vi "rightJustifyColumn.vi"(8 "error in (no error)":errorcluster, 11 "ScriptEditorV2 in":refnum<class "ScriptEditorV2.lvclass">) -> (0 "error out":errorcluster, 3 "ScriptEditorV2 out":refnum<class "ScriptEditorV2.lvclass">)   [LabVIEW 2011, in "Views.lvlib" / "ScriptEditor.lvlib" / "ScriptEditorV2.lvclass"]
uses:
  ScriptEditorV2.lvclass
  ScriptEditorV2.lvclass/ScriptEditorV2.ctl
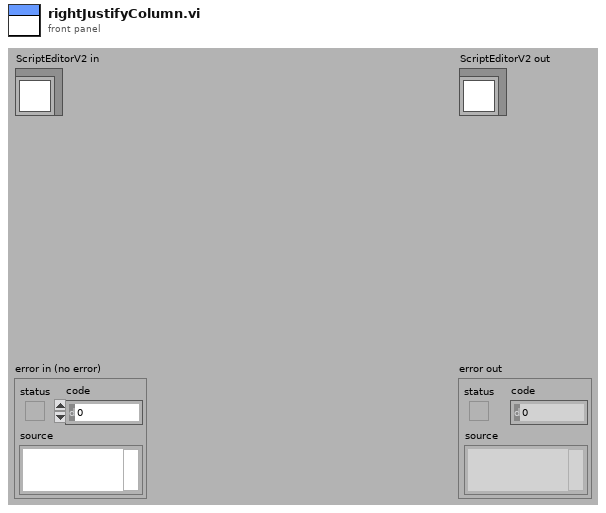
[diagram p1: front panel]
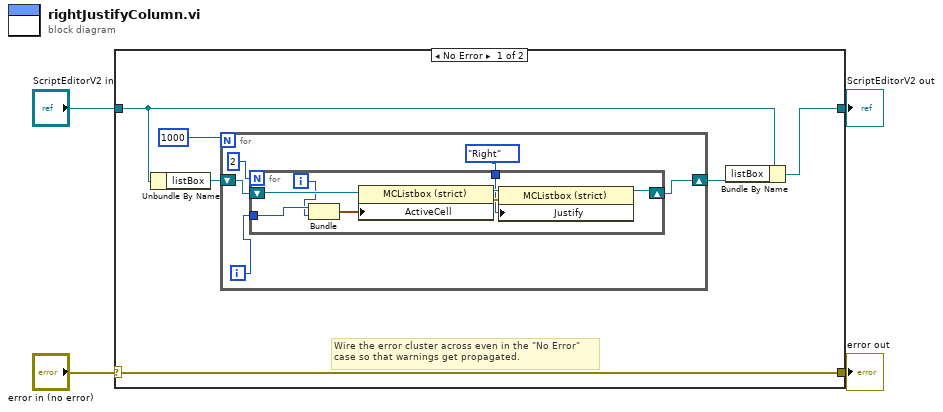
[diagram p0: block diagram]
diagram:
  n1 = case shown="No Error" "error in (no error)" {
    selector: "error in (no error)" -> [w10 w25]
    tunnel: [w10 w25] -> w3
    tunnel: [w6 w24] -> w1
    tunnel: "ScriptEditorV2 in" -> [w7 w24]
    frame No Error {
      # "Wire the error cluster across even in the \"No Error\"\ncase so that warnings get propagated."
      n2 = Unbundle By Name(w7) -> ("listBox"=w9:refnum<vi>)
      n3 = for {
        N: 1000 -> [_]
        shift-right: [w14] -> w8
        shift-left: w9 -> [w15]
        i -> [w13]
        n4 = for {
          N: 2 -> [_]
          tunnel: w13 -> [w17]
          shift-right: [w20] -> w14
          shift-left: w15 -> [w23]
          tunnel: enum16{"Left", "Center", "Right"}."Right" ("Active Cell:Cell Justification") -> [w18]
          i -> [w16]
          n5 = Bundle(w17, w16) -> (w22:cluster{i32, i32})  [unwired: 1 in]
          n6 = property class="MCListbox (strict)"(reference=w23, "ActiveCell"=w22) -> (reference out=w21:refnum<vi>, error out=w19:errorcluster)  [unwired: 1 in]
          n7 = property class="MCListbox (strict)"(reference=w21, error in=w19, "Justify"=w18) -> (reference out=w20:refnum<vi>)  [unwired: 1 out]
        }
      }
      n8 = Bundle By Name(cluster=w7, "listBox"=w8) -> (w6:refnum<class "ScriptEditorV2.lvclass">)
    }
    frame Error {
    }
  }
  "error out" <- w3
  "ScriptEditorV2 out" <- w1
